vi "GetBlockquoteTag.vi"(8 "error in (no error)":errorcluster, 11 "Blockquote in":refnum<class "Blockquote.lvclass">) -> (0 "error out":errorcluster, 2 "BlockquoteTag":string, 3 "Blockquote out":refnum<class "Blockquote.lvclass">)   [LabVIEW 2021, in "LvMarkdown.lvlib" / "Blockquote.lvclass"]
uses:
  Blockquote.lvclass
  Blockquote.lvclass/Blockquote.ctl
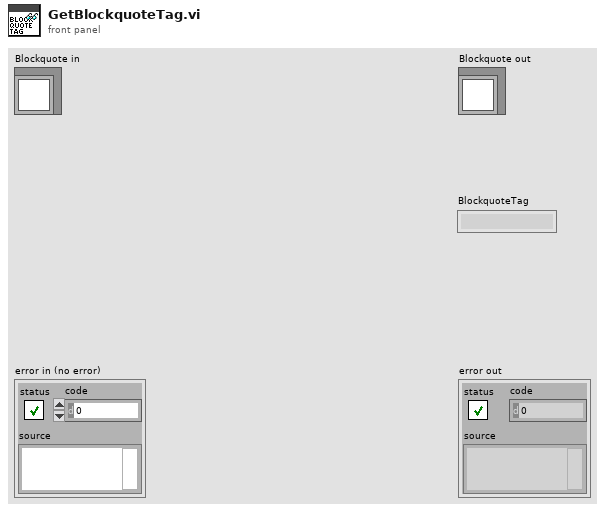
[diagram p1: front panel]
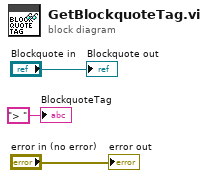
[diagram p0: block diagram]
diagram:
  "error out" <- "error in (no error)"
  "Blockquote out" <- "Blockquote in"
  "BlockquoteTag" <- "> " ("BlockquoteTag")
